vi "BundleAutoSpotDataIngoHeucke.vi"(2 "auto":bool, 3 "notes 2":refnum<vi>, 4 "already x spots":i16, 5 "Enum":enum16{"1st sort", "Display", "Get"}(ring)) -> (1 "Spots out":T1[](array[typedef]) {"F2-Value overall" format="%.2f"; "tauerror" format="%.2f"; "Lifetime[ns]" format="%.2f"; "F2-Value TAC" format="%.2f"})   [LabVIEW 2009]
uses:
  spotproperties.ctl
  <vilib>/vision/NI_Vision_Development_Module.lvlib
panel:
  in  "draw?":bool
  in  "notes":string
  out "F2-Value overall":sgl format="%.2f"
  in  "Ring":u16(ring) items=["linear y-axis", "log y-axis"]
  in  "stop":bool
  out "TAC intensity":u32[](array[numeric])
  out "overall intensity":u32[](array[numeric])
  out "tauerror [ns]":dbl[](array[numeric]) format="%.2f"
  out "Lifetime [ns]":ext[](array[numeric]) format="%.2f"
  out "F2-Value TAC":dbl format="%.2f"
  in  "SpotNo.":u16 min=36 max=70
  out "Decays":u32[][](graph)
  # "S"
  # "S"
  # "S"
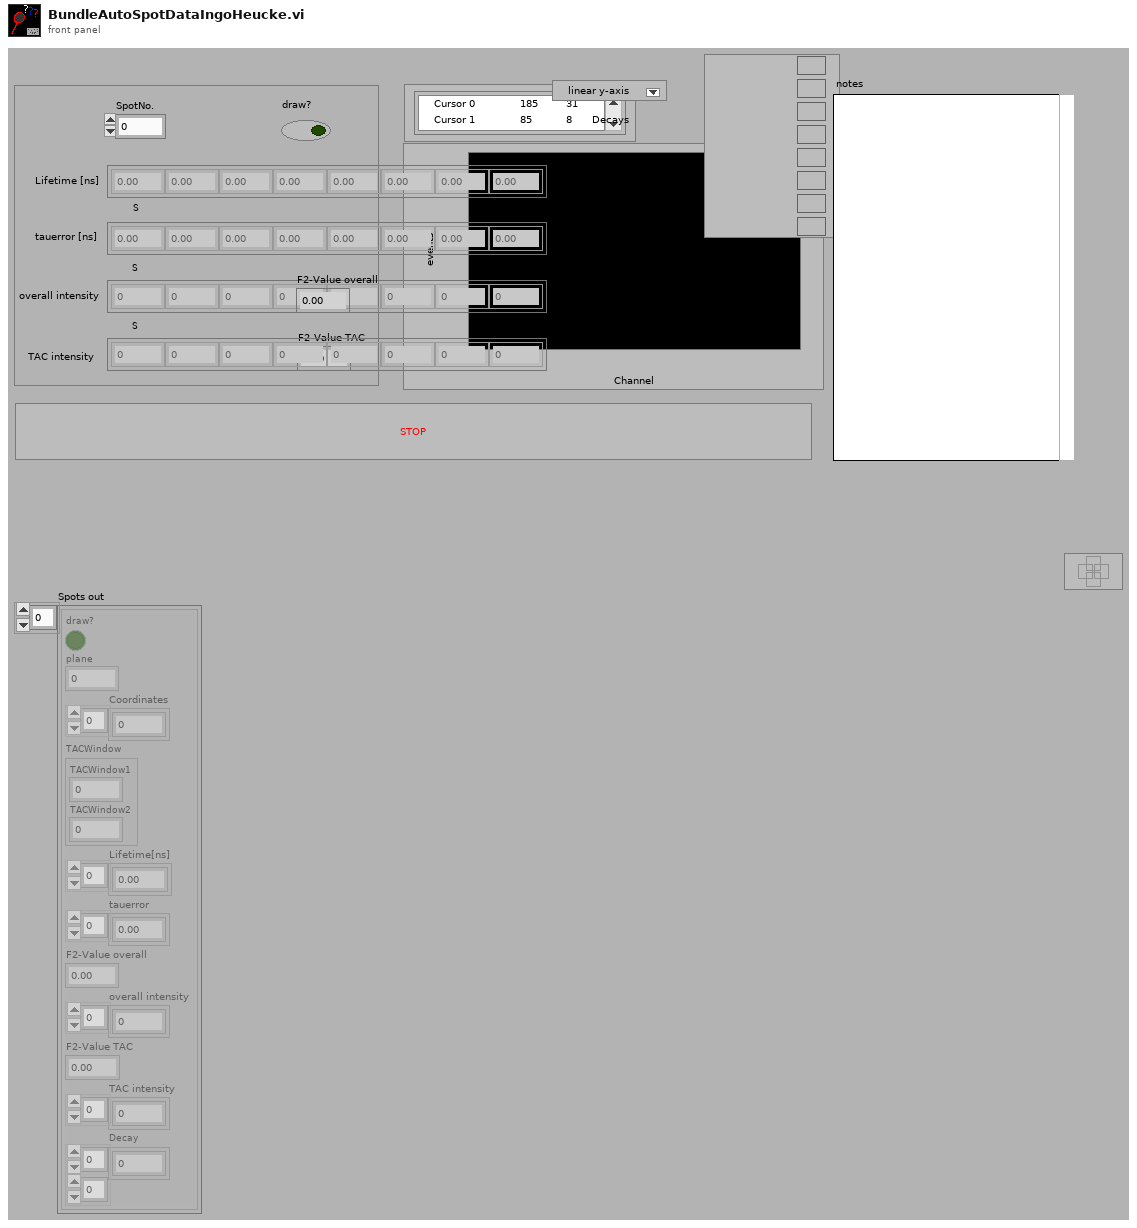
[diagram p1: front panel]
types:
  T1 = typedef "spotproperties.ctl" = cluster{"draw?":bool, "plane":u32, "Coordinates":i32[], "TACWindow":cluster{"TACWindow1":i32, "TACWindow2":i32}, "Lifetime[ns]":ext[], "tauerror":dbl[], "F2-Value overall":dbl, "overall intensity":u32[], "F2-Value TAC":dbl, "TAC intensity":u32[], "Decay":u32[][]}
  T2 = enum16{"Ini", "Get", "Set", "Refresh", "dump", "move", "name"}
  T3 = typedef "Settings.ctl" = cluster{"threshold":cluster{"max":u32, "min":u32}, "RGB or false color":bool, "16bit":bool, "log/lin axis":u16, "spotsize button":bool, "Pixelsize":u16, "autoscale x":bool, "autoscale y":bool, "correlation":bool, "ADC-Resolution":i32, "F2-lifetime":cluster{"display tau":bool, "display F2":bool, "Palette Number lifetime":enum32{"Gray", "Binary", "Gradient", "Rainbow", "Temperature"}, "Palette Number F2":enum32{"Gray", "Binary", "Gradient", "Rainbow", "Temperature"}, "max tau-Value":dbl, "min tau-Value":dbl, "max F2-Value":dbl, "min F2-Value":dbl}, "TAC-Window 1":u16, "TAC-Window 2":u16, "false color palette":cluster{"1":u32, "2":u32, "3":u32, "4":u32, "5":u32, "6":u32, "7":u32, "8":u32, "8 2":u32, "8 3":u32, "8 4":u32, "8 5":u32}}
  T4 = typedef "IMAQ Image.ctl" = refnum<image>
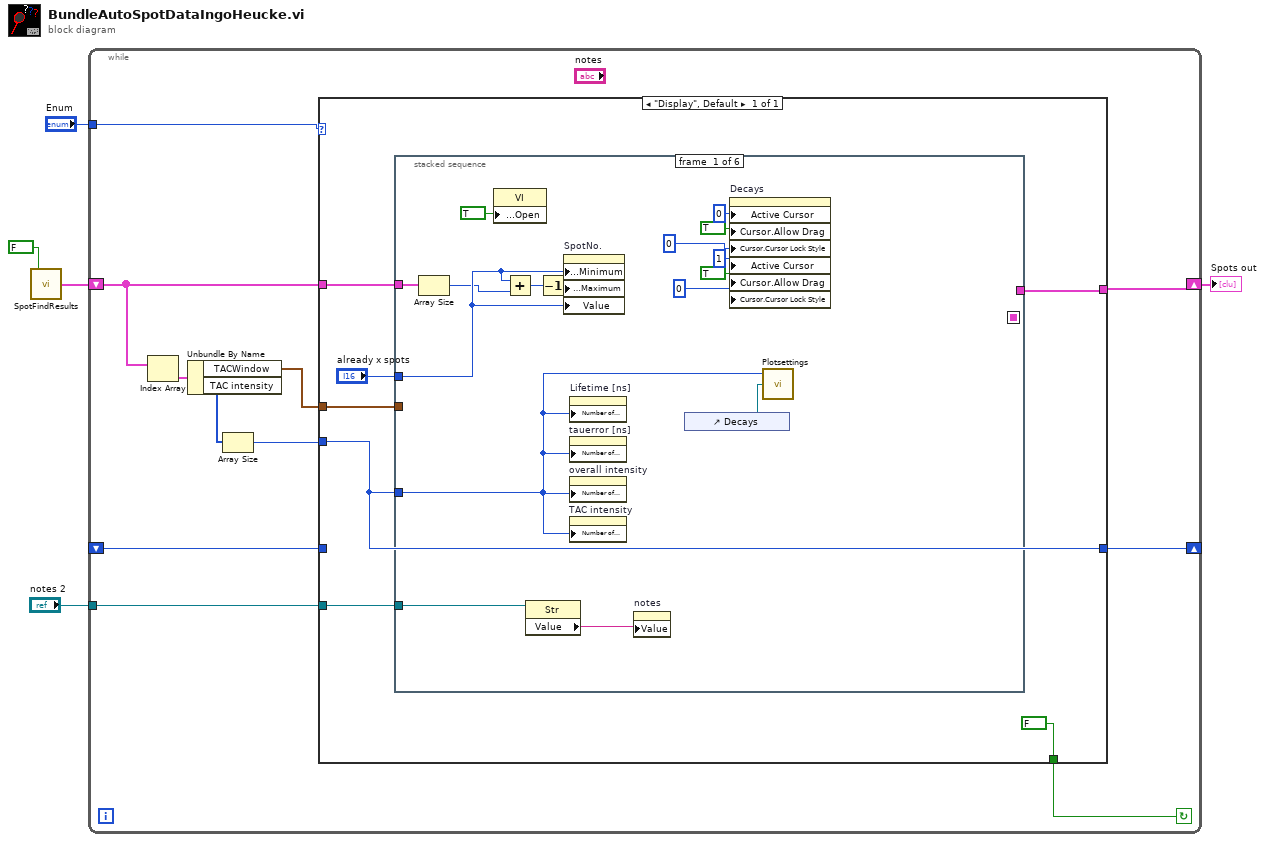
[diagram p0: block diagram]
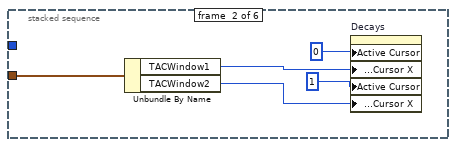
[diagram p2: hidden frame]
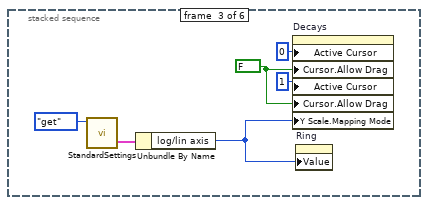
[diagram p3: hidden frame]
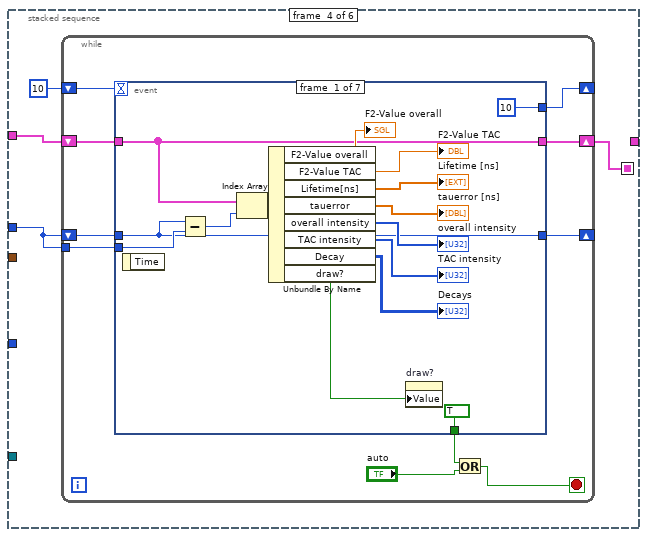
[diagram p4: hidden frame]
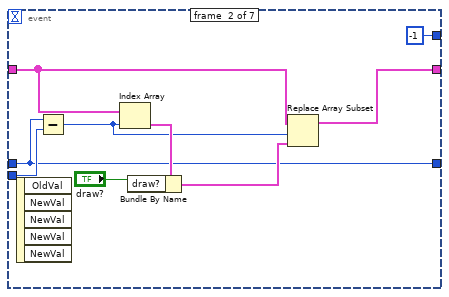
[diagram p5: hidden frame]
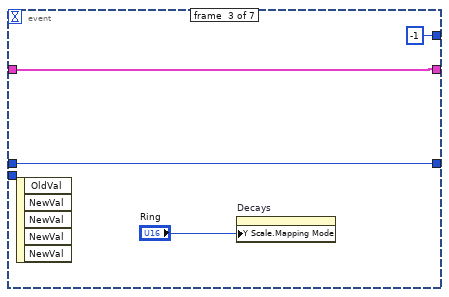
[diagram p6: hidden frame]
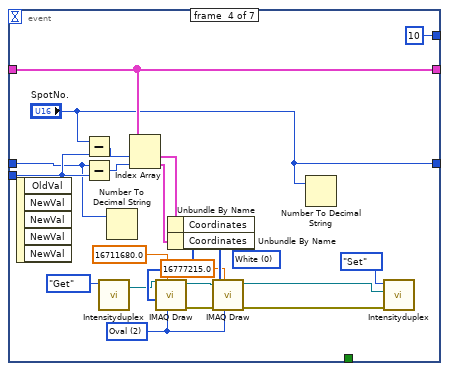
[diagram p7: hidden frame]
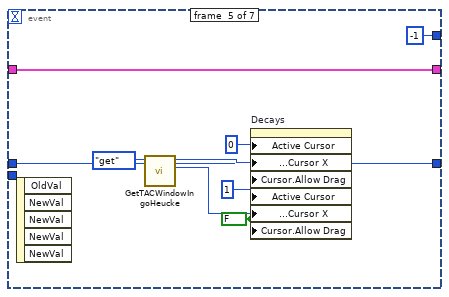
[diagram p8: hidden frame]
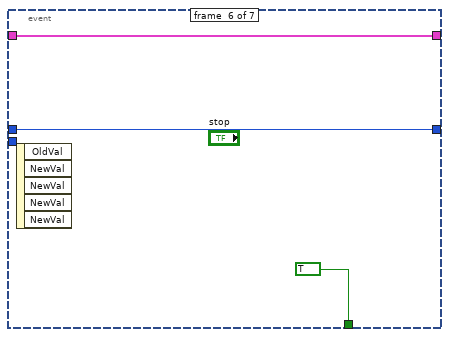
[diagram p9: hidden frame]
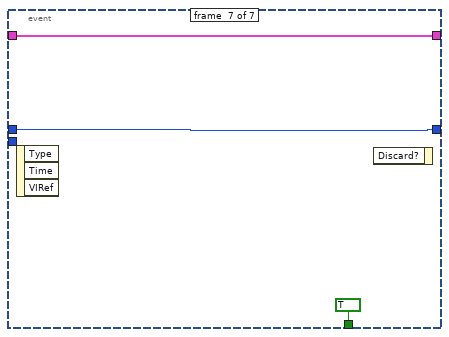
[diagram p10: hidden frame]
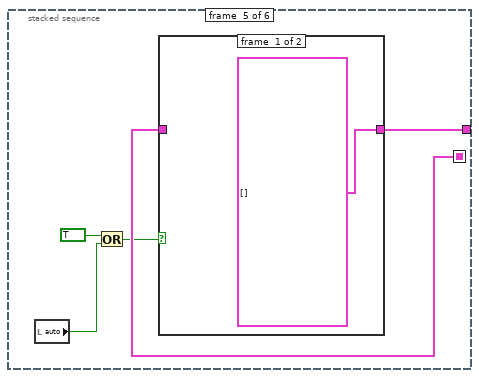
[diagram p11: hidden frame]
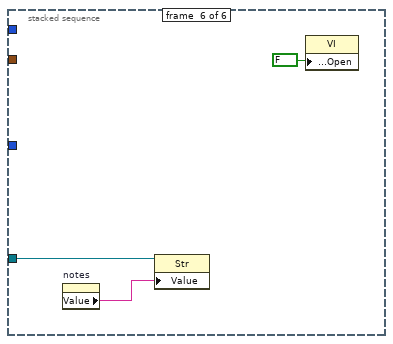
[diagram p13: hidden frame]
diagram:
  n1 = call "SpotFindResults.vi"("set?"=FALSE) -> ("Spots out"=w4:T1[])  [unwired: 4 in]
  n2 = while {
    shift-right: [w15] -> w1
    shift-left: w4 -> [w12]
    shift-right: [w14] -> _
    shift-left: _ -> [w13]
    tunnel: "Enum" -> [w7]
    tunnel: "notes 2" -> [w6]
    stop <- w16 continue-if-true
    n3 = Index Array(array=w12) -> (element=w11:T1)  [unwired: 1 in]
    n4 = Unbundle By Name(w11) -> ("TACWindow"=w10:cluster{"TACWindow1":i32, "TACWindow2":i32}, "TAC intensity"=w9:u32[])
    n5 = Array Size(array=w9) -> (size(s)=w8:i32)
    n6 = case shown="\"Display\", Default" w7 {
      tunnel: [FALSE] -> w16
      tunnel: [w22] -> w15
      tunnel: w12 -> [w23]
      tunnel: [w19] -> w14
      tunnel: w13 -> [_]
      tunnel: w10 -> [w20]
      tunnel: w8 -> [w19]
      tunnel: w6 -> [w17]
      frame "Display", Default {
        n7 = stacked-sequence {
          seq-local: [_ _ _ w52 _ _] -> [_ _ _ _ w132 _]
          tunnel: w23 -> [w38 _ _ w53 _ _]
          tunnel: [_ _ _ _ w133 _] -> w22
          tunnel: w19 -> [w28 _ _ _ _ _]
          tunnel: "already x spots" -> [w27 _ _ w51 _ _]
          tunnel: w20 -> [_ w42 _ _ _ _]
          tunnel: w17 -> [w30 _ _ _ _ w136]
          frame #0 {
            n8 = Array Size(array=w38) -> (size(s)=w26:i32)
            n9 = property class="VI"("Front Panel Window:Open"=TRUE) -> ()  [unwired: 2 in, 2 out]
            n10 = Add(x=w27, y=w26) -> (x+y=w25:i32)
            n11 = property class="Str"(reference=w30) -> ("Value"=w31:string)  [unwired: 1 in, 2 out]
            n12 = Decrement(x=w25) -> (x-1=w24:i32)
            n13 = property on="SpotNo." class="Digital (strict)"("Data Entry Limits:Minimum"=w27, "Data Entry Limits:Maximum"=w24, "Value"=w27) -> ()  [unwired: 2 in, 2 out]
            n14 = property on="Lifetime [ns]" class="Arr (strict)"("Number of Columns"=w28) -> ()  [unwired: 2 in, 2 out]
            n15 = property on="tauerror [ns]" class="Arr (strict)"("Number of Columns"=w28) -> ()  [unwired: 2 in, 2 out]
            n16 = property on="overall intensity" class="Arr (strict)"("Number of Columns"=w28) -> ()  [unwired: 2 in, 2 out]
            n17 = property on="TAC intensity" class="Arr (strict)"("Number of Columns"=w28) -> ()  [unwired: 2 in, 2 out]
            n18 = property on="notes" class="String"("Value"=w31) -> ()  [unwired: 2 in, 2 out]
            n19 = control-ref of="Decays"() -> (w29:refnum<vi>)
            n20 = property on="Decays" class="WFGraph (strict)"("Active Cursor"=u32 0, "Cursor.Allow Drag"=TRUE, "Cursor.Cursor Lock Style"=u32 0 ("Cursor.Cursor Locked"), "Active Cursor"=u32 1, "Cursor.Allow Drag"=TRUE, "Cursor.Cursor Lock Style"=u32 0 ("Cursor.Cursor Locked")) -> ()  [unwired: 2 in, 2 out]
            n21 = call "Plotsettings.vi"("Decays 2"=w29, "No of Channels"=w28) -> ()  [unwired: 4 in]
          }
          frame #1 {
            n22 = Unbundle By Name(w42) -> ("TACWindow1"=w41:i32, "TACWindow2"=w40:i32)
            n23 = property on="Decays" class="WFGraph (strict)"("Active Cursor"=u32 0, "Cursor.Cursor Position:Cursor X"=w41, "Active Cursor"=u32 1, "Cursor.Cursor Position:Cursor X"=w40) -> ()  [unwired: 2 in, 2 out]
          }
          frame #2 {
            w50 = FALSE ("Cursor.Allow Drag")
            n24 = call "StandardSettings.vi"("Enum"=enum16{"Load", "get", "Save", "set"}."get") -> ("StandardSettings"=w46:T3)  [unwired: 4 in]
            n25 = Unbundle By Name(w46) -> ("log/lin axis"=w45:u16)
            n26 = property on="Decays" class="WFGraph (strict)"("Active Cursor"=u32 0, "Cursor.Allow Drag"=w50, "Active Cursor"=u32 1, "Cursor.Allow Drag"=w50, "Y Scale.Mapping Mode"=w45) -> ()  [unwired: 2 in, 2 out]
            n27 = property on="Ring" class="Ring (strict)"("Value"=w45) -> ()  [unwired: 2 in, 2 out]
          }
          frame #3 {
            n28 = while {
              shift-right: [w61] -> _
              shift-left: 10 -> [w62]
              shift-right: [w64] -> _
              shift-left: w51 -> [w63]
              shift-right: [w60] -> w52
              shift-left: w53 -> [w59]
              tunnel: w51 -> [w58]
              stop <- w55 stop-if-true
              n29 = event shown="[4] \"Decays\": Value Change" {
                selector: _ -> [_ _ _ _ _ _ _]
                dyn-events: _ -> [_ _ _ _ _ _ _]
                timeout: w62 -> [_ _ _ _ _ _ _]
                tunnel: w59 -> [w69 w88 w90 w110 w116 w124 w127]
                tunnel: [TRUE _ _ _ _ TRUE TRUE] -> w57
                tunnel: [w66 w81 w89 "SpotNo." w115 w123 w126] -> w64
                tunnel: w63 -> [w66 w81 w89 w101 w115 w123 w126]
                tunnel: [10 -1 -1 10 -1 _ _] -> w61
                tunnel: [w69 w85 w90 w110 w116 w124 w127] -> w60
                tunnel: w58 -> [w68 w82 _ w111 _ _ _]
                event #0 {
                  n30 = event-data() -> ()  [unwired: 1 in, 1 out]
                  n31 = Subtract(x=w66, y=w68) -> (x-y=w67:u16)
                  n32 = Index Array(array=w69, index=w67) -> (element=w79:T1)
                  n33 = Unbundle By Name(w79) -> ("F2-Value overall"=→"F2-Value overall":dbl, "F2-Value TAC"=→"F2-Value TAC":dbl, "Lifetime[ns]"=→"Lifetime [ns]":ext[], "tauerror"=→"tauerror [ns]":dbl[], "overall intensity"=→"overall intensity":u32[], "TAC intensity"=→"TAC intensity":u32[], "Decay"=→"Decays":u32[][], "draw?"=w70:bool)
                  n34 = property on="draw?" class="Boolean (strict)"("Value"=w70) -> ()  [unwired: 2 in, 2 out]
                }
                event #1 {
                  n35 = event-data() -> ()  [unwired: 1 in, 5 out]
                  n36 = Subtract(x=w81, y=w82) -> (x-y=w80:u16)
                  n37 = Index Array(array=w88, index=w80) -> (element=w87:T1)
                  n38 = Bundle By Name(cluster=w87, "draw?"="draw?") -> (w86:T1)
                  n39 = Replace Array Subset(array=w88, new element=w86, index=w80) -> (w85:T1[])
                }
                event #2 {
                  n40 = event-data() -> ()  [unwired: 1 in, 5 out]
                  n41 = property on="Decays" class="WFGraph (strict)"("Y Scale.Mapping Mode"="Ring") -> ()  [unwired: 2 in, 2 out]
                }
                event #3 {
                  (unwired) 0 items=["White", "Black", "Inverted", "Black on White", "White on Black"] ("Color")
                  w106 = u16 2 items=["Line", "Rectangle", "Oval"] ("Shape to draw")
                  n42 = event-data() -> ()  [unwired: 1 in, 5 out]
                  n43 = Subtract(x="SpotNo.", y=w111) -> (x-y=w109:u16)
                  n44 = Subtract(x=w101, y=w111) -> (x-y=w102:u16)
                  n45 = call "Intensityduplex.vi"("Enum"=T2."Get") -> ("Image Duplicate (out)"=w96:T4)  [unwired: 4 in, 1 out]
                  n46 = Number To Decimal String(number=w101) -> ()  [unwired: 1 in, 1 out]
                  n47 = Index Array(array=w110, index #1=w109, index #2=w102) -> (element #1=w107:T1, element #2=w108:T1)
                  n48 = Unbundle By Name(w107) -> ("Coordinates"=w103:i32[])
                  n49 = call "IMAQ Draw"("Shape to draw"=w106, "Pixel Color"=sgl 16711680.0, "Coordinates"=w103, "Image Src"=w96) -> ("error out"=w104:errorcluster, "Image Dst Out"=w95:T4)  [unwired: 6 in]
                  n50 = Unbundle By Name(w108) -> ("Coordinates"=w99:i32[])
                  n51 = call "IMAQ Draw"("Shape to draw"=w106, "Pixel Color"=sgl 16777215.0, "error in (no error)"=w104, "Coordinates"=w99, "Image Src"=w95) -> ("error out"=w93:errorcluster, "Image Dst Out"=w94:T4)  [unwired: 5 in]
                  n52 = Number To Decimal String(number="SpotNo.") -> ()  [unwired: 1 in, 1 out]
                  n53 = call "Intensityduplex.vi"("Enum"=T2."Set", "Image In"=w94, "error in"=w93) -> ()  [unwired: 2 in, 2 out]
                }
                event #4 {
                  w117 = FALSE ("Cursor.Allow Drag")
                  n54 = event-data() -> ()  [unwired: 1 in, 5 out]
                  n55 = call "GetTACWindowIngoHeucke.vi"("Enum"=enum16{"ini", "get", "quick"}."get") -> ("Cursor.Cursor Position:Cursor X"=w121:u16, "Cursor.Cursor Position:Cursor X 2"=w120:u16)  [unwired: 1 in, 7 out]
                  n56 = property on="Decays" class="WFGraph (strict)"("Active Cursor"=u32 0, "Cursor.Cursor Position:Cursor X"=w121, "Cursor.Allow Drag"=w117, "Active Cursor"=u32 1, "Cursor.Cursor Position:Cursor X"=w120, "Cursor.Allow Drag"=w117) -> ()  [unwired: 2 in, 2 out]
                }
                event #5 {
                  n57 = event-data() -> ()  [unwired: 1 in, 5 out]
                }
                event #6 {
                  n58 = event-data() -> ()  [unwired: 1 in, 3 out]
                  n59 = event-data() -> ()  [unwired: 2 in, 1 out]
                }
              }
              n60 = Or(x=w57, y="auto") -> (x .or. y?=w55:bool)
            }
          }
          frame #4 {
            n61 = local read "auto"() -> (w131:bool)
            n62 = Or(x=TRUE, y=w131) -> (x .or. y?=w130:bool)
            n63 = case shown="True" w130 {
              tunnel: w132 -> [_ w135]
              tunnel: [T1[] [] ("Spots out") w135] -> w133
              frame #0 {
              }
              frame #1 {
              }
            }
          }
          frame #5 {
            n64 = property on="notes" class="String"() -> ("Value"=w137:string)  [unwired: 2 in, 2 out]
            n65 = property class="Str"(reference=w136, "Value"=w137) -> ()  [unwired: 1 in, 2 out]
            n66 = property class="VI"("Front Panel Window:Open"=FALSE) -> ()  [unwired: 2 in, 2 out]
          }
        }
      }
    }
  }
  "Spots out" <- w1
